vi "19572_read_PASS_FAIL_status.vi"(8 "error in (no error)":errorcluster, 10 "timeout":dbl=10.0 format="%0.2f", 11 "task/channels in":refnum<k21>) -> (0 "error out":errorcluster, 1 "Fail":bool, 2 "Pass":bool, 3 "task out":refnum<k21>)   [LabVIEW 2015]
uses:
  <vilib>/DAQmx/read.llb/DAQmx Read (Digital 1D Bool 1Chan 1Samp).vi
  <vilib>/DAQmx/miscellaneous.llb/DAQmx Fill In Error Info.vi
panel:
  # "Read CHROMA 19572 FAIL & PASS LEDs status"
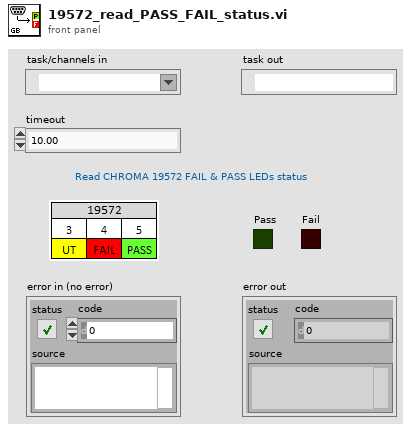
[diagram p1: front panel]
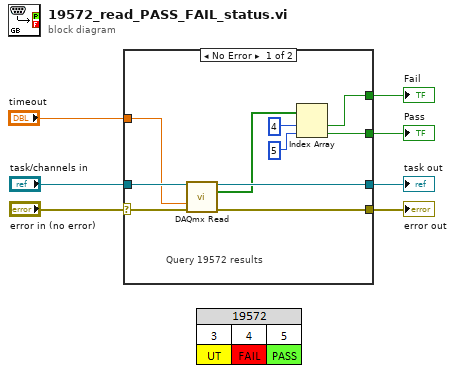
[diagram p0: block diagram]
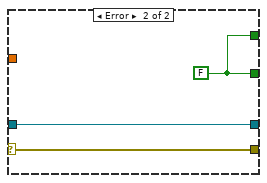
[diagram p2: hidden frame]
diagram:
  n1 = case shown="No Error" "error in (no error)" {
    selector: "error in (no error)" -> [w9 w19]
    tunnel: "task/channels in" -> [w15 w20]
    tunnel: [w14 w20] -> w6
    tunnel: [w13 w18] -> w5
    tunnel: [w12 w18] -> w4
    tunnel: [w11 w19] -> w3
    tunnel: "timeout" -> [w8 _]
    frame No Error {
      # "Query 19572 results"
      n2 = call-poly <vilib>:"DAQmx Read.vi"("task/channels in"=w15, "timeout"=w8, "error in"=w9) -> ("task out"=w14:refnum<k21>, "data"=w10:bool[], "error out"=w11:errorcluster)  [unwired: 10 in]
      n3 = Index Array(array=w10, index #1=4 ("index"), index #2=5 ("index")) -> (element #1=w13:bool, element #2=w12:bool)
    }
    frame Error {
      w18 = FALSE
    }
  }
  "task out" <- w6
  "error out" <- w3
  "Fail" <- w5
  "Pass" <- w4
